vi "Position miniscan index number on image.vi"(11 "X-Y-Z coordinates":T1 {"ROI group ID" format="%#_6f"; "Laser Power (%)" format="%#_6f"; "Zoom" format="%#_6f"; "Frame Size" format="%#_6f"; "Number of lines" format="%#_6f"; "Composite ID" format="%#_6f"; "Angle (deg)" format="%#_6f"; "ROI Time (ns)" format="%#_6f"; "ROI ID" format="%#_6f"; "Pixels in ROI" format="%#_6f"; "ROI index" format="%#_6f"; "Z stop" format="%#_6f"; "Y stop" format="%#_6f"; "X stop" format="%#_6f"; "Z start" format="%#_6f"; "X start" format="%#_6f"; "Y start" format="%#_6f"}) -> (1 "X-Y coordinates at miniscan middle point":cluster{"X":i32, "Y":i32})   [LabVIEW 2017]
uses:
  Typedefs/ROI parameters data type.ctl
panel:
  in  "Fixed Y-axis offset (pixels)":i32=-1
  in  "Fixed X-axis offset (pixels)":i32
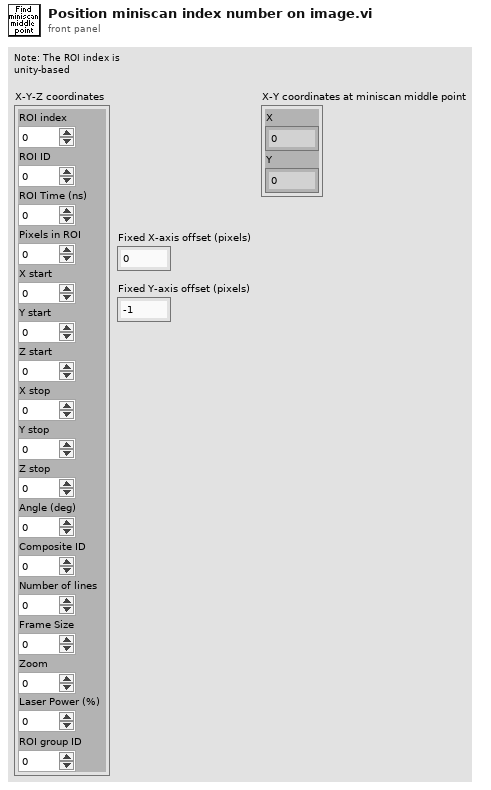
[diagram p1: front panel]
types:
  T1 = typedef "ROI parameters data type.ctl" = cluster{"ROI index":dbl, "ROI ID":dbl, "ROI Time (ns)":dbl, "Pixels in ROI":dbl, "X start":dbl, "Y start":dbl, "Z start":dbl, "X stop":dbl, "Y stop":dbl, "Z stop":dbl, "Angle (deg)":dbl, "Composite ID":dbl, "Number of lines":dbl, "Frame Size":dbl, "Zoom":dbl, "Laser Power (%)":dbl, "ROI group ID":dbl}
  T2 = enum16{"ID to the left of miniscan", "ID to the top of miniscan"}
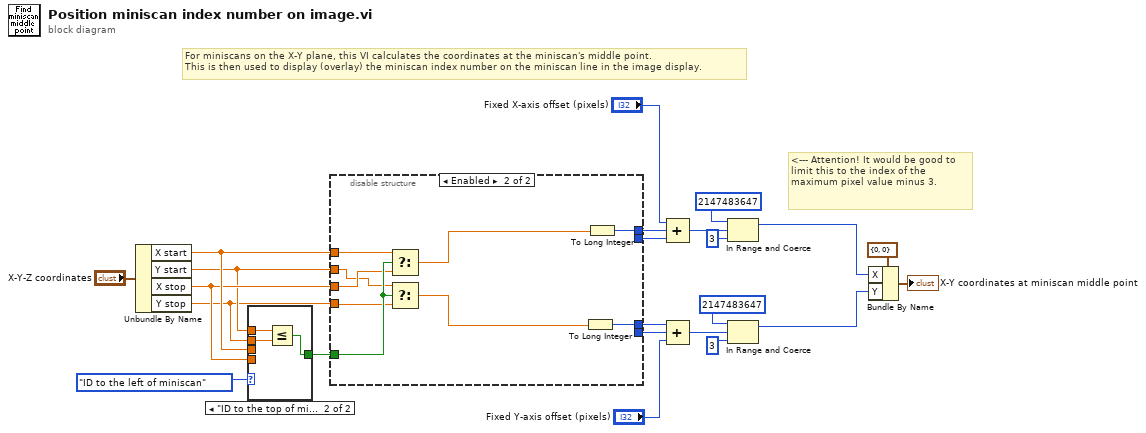
[diagram p0: block diagram]
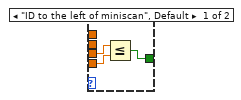
[diagram p2: hidden frame]
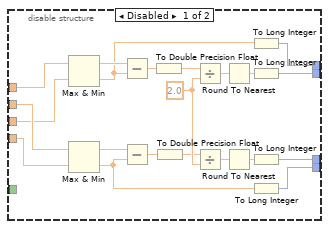
[diagram p3: hidden frame]
diagram:
  # "<--- Attention! It would be good to limit this to the index of the maximum pixel value minus 3."
  # "For miniscans on the X-Y plane, this VI calculates the coordinates at the miniscan's middle point.\nThis is then used to display (overlay) the miniscan index number on the miniscan line in the image display."
  n1 = Unbundle By Name("X-Y-Z coordinates") -> ("X start"=w5:dbl, "Y start"=w2:dbl, "X stop"=w4:dbl, "Y stop"=w1:dbl)
  n2 = case shown="\"ID to the top of miniscan\"" T2."ID to the left of miniscan" ("Enum") {
    tunnel: [w26 w27] -> w6
    tunnel: w5 -> [w25 _]
    tunnel: w4 -> [w24 _]
    tunnel: w2 -> [_ w29]
    tunnel: w1 -> [_ w28]
    frame "ID to the left of miniscan", Default {
      n3 = Less Or Equal?(x=w25, y=w24) -> (x <= y?=w26:bool)
    }
    frame "ID to the top of miniscan" {
      n4 = Less Or Equal?(x=w29, y=w28) -> (x <= y?=w27:bool)
    }
  }
  n5 = disable-structure shown="Enabled" {
    disable-tunnel: w1 -> [w46 w56]
    disable-tunnel: w2 -> [w45 w51]
    disable-tunnel: w4 -> [w44 w55]
    disable-tunnel: w5 -> [w43 w53]
    disable-tunnel: [w35 _] -> w20
    disable-tunnel: [w34 _] -> w19
    disable-tunnel: [w33 w59] -> w18
    disable-tunnel: [w32 w58] -> w17
    disable-tunnel: w6 -> [_ w57]
    frame Disabled {
      w42 = 2.0 ("y")
      n6 = Max & Min(x=w43, y=w44) -> (max(x,y)=w36:dbl, min(x,y)=w31:dbl)
      n7 = Max & Min(x=w45, y=w46) -> (max(x,y)=w37:dbl, min(x,y)=w30:dbl)
      n8 = Subtract(x=w36, y=w31) -> (x-y=w38:dbl)
      n9 = Subtract(x=w37, y=w30) -> (x-y=w40:dbl)
      n10 = To Double Precision Float(number=w38) -> (double precision float=w39:dbl)
      n11 = To Double Precision Float(number=w40) -> (double precision float=w41:dbl)
      n12 = Divide(x=w39, y=w42) -> (x/y=w47:dbl)
      n13 = Divide(x=w41, y=w42) -> (x/y=w49:dbl)
      n14 = Round To Nearest(number=w47) -> (nearest integer value=w48:dbl)
      n15 = Round To Nearest(number=w49) -> (nearest integer value=w50:dbl)
      n16 = To Long Integer(number=w31) -> (32bit integer=w33:i32)
      n17 = To Long Integer(number=w48) -> (32bit integer=w34:i32)
      n18 = To Long Integer(number=w50) -> (32bit integer=w32:i32)
      n19 = To Long Integer(number=w30) -> (32bit integer=w35:i32)
    }
    frame Enabled {
      n20 = Select(t=w53, s=w57, f=w55) -> (s? t:f=w52:dbl)
      n21 = Select(t=w51, s=w57, f=w56) -> (s? t:f=w54:dbl)
      n22 = To Long Integer(number=w54) -> (32bit integer=w58:i32)
      n23 = To Long Integer(number=w52) -> (32bit integer=w59:i32)
    }
  }
  n24 = Compound Arithmetic op=ADD("Fixed X-axis offset (pixels)", w18, w19) -> (w13:i32)
  n25 = Compound Arithmetic op=ADD(w17, w20, "Fixed Y-axis offset (pixels)") -> (w16:i32)
  n26 = In Range and Coerce(upper limit=2147483647, x=w13, lower limit=3) -> (coerced(x)=w8:i32)  [unwired: 1 out]
  n27 = In Range and Coerce(upper limit=2147483647, x=w16, lower limit=3) -> (coerced(x)=w7:i32)  [unwired: 1 out]
  n28 = Bundle By Name(cluster=cluster{"X":i32, "Y":i32} {"X"=0, "Y"=0} ("Point"), "X"=w8, "Y"=w7) -> (→"X-Y coordinates at miniscan middle point":cluster{"X":i32, "Y":i32})
